vi "Set Event.vi"(8 "error in (no error)":errorcluster, 10 "Event name":string, 11 "Event in":refnum<class "Event.lvclass">) -> (0 "error out":errorcluster, 3 "Event out":refnum<class "Event.lvclass">)   [LabVIEW 2013, in "MDSplus.lvlib" / "Event.lvclass"]
doc: "Issues a new event."
uses:
  <vilib>/MDSplus/Classes/Event_Class/Event.lvclass
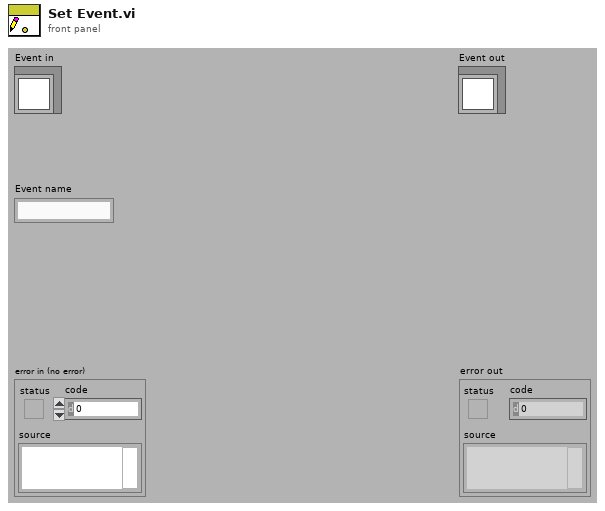
[diagram p1: front panel]
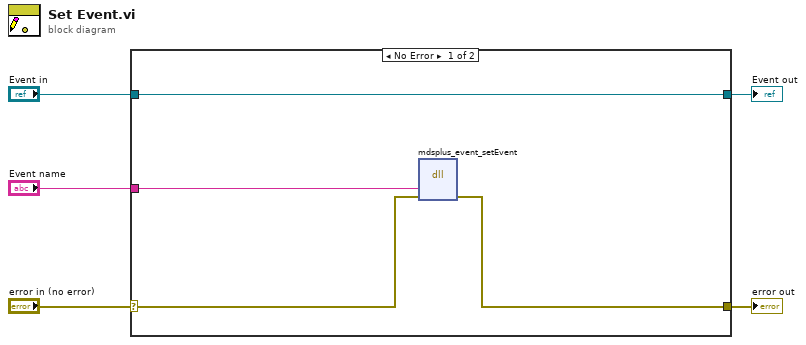
[diagram p0: block diagram]
diagram:
  n1 = case shown="No Error" "error in (no error)" {
    selector: "error in (no error)" -> [w8 w10]
    tunnel: [w7 w10] -> w4
    tunnel: [w6 w11] -> w3
    tunnel: "Event in" -> [w6 w11]
    tunnel: "Event name" -> [w9 _]
    frame No Error {
      n2 = dll-call lib="MDSobjectsLVShr" fn="mdsplus_event_setEvent"("evNameIn"=w9, "error"=w8) -> ("error"=w7:errorcluster)  [unwired: 5 in, 2 out]
    }
    frame Error {
    }
  }
  "error out" <- w4
  "Event out" <- w3
